vi "mqttTCPIPserver.vi"(0 "mqtt.lvclass":refnum<class "mqtt.lvclass">, 11 "error in (no error)":errorcluster) -> (4 "mqtt.lvclass 2":refnum<class "mqtt.lvclass">, 15 "error out":errorcluster)   [LabVIEW 2013, in "mqtt.lvclass"]
uses:
  mqtt.lvclass
  mqttTXqueue/mqttTXdataQueueFunction.ctl
  mqttTypedef/mqttQOSlevel.ctl
  mqttTypedef/mqttMessageType.ctl
  mqttTypedef/mqttFixedHeaderResponse.ctl
  mqttTypedef/mqttRXdataCluster.ctl
  mqttTXqueue/mqttRXsubscriptionEventFunction.ctl
  mqttTXqueue/mqttRXsubscriptionEventData.ctl
panel:
  out "rxCount":i32
  out "rxTelegram":u8[](array[numeric]) format="%02x"
  out "txError":errorcluster
  out "txTelegram":u8[](array[numeric]) format="%02x"
  out "payloadError":errorcluster
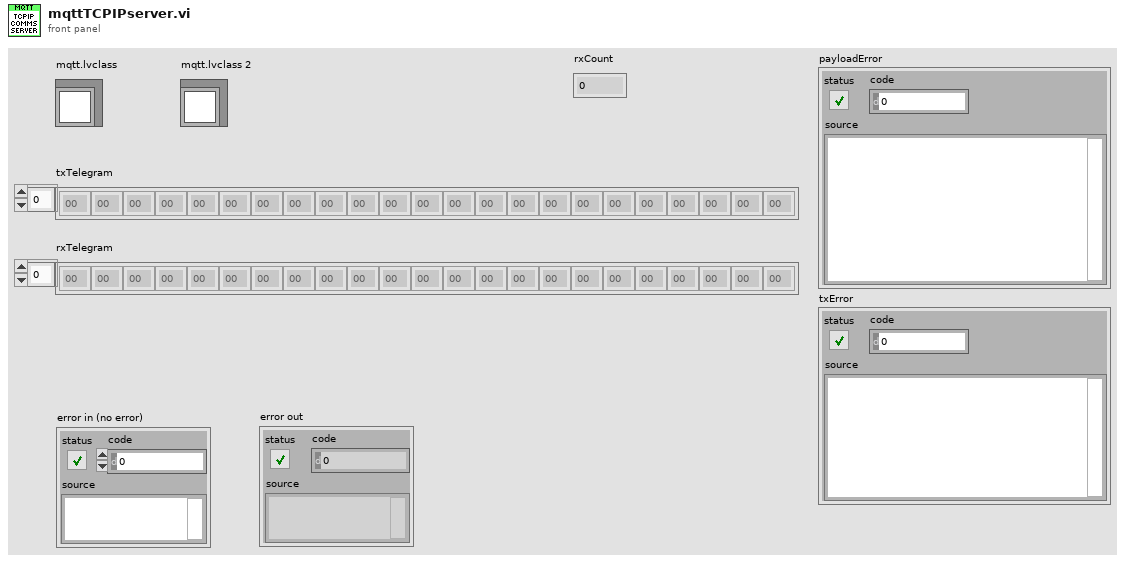
[diagram p1: front panel]
types:
  T1 = typedef "mqttTXdataQueueFunction.ctl" = enum16{"init", "deinit", "getQueue", "enqueue"}
  T2 = typedef "mqttRXdataCluster.ctl" = cluster{"fixedHdr":T3, "payload":u8[]}
  T3 = typedef "mqttFixedHeaderResponse.ctl" = cluster{"retain":bool, "qos":T4, "duplicate":bool, "response":T5}
  T4 = typedef "mqttQOSlevel.ctl" = enum8{"At most once", "At least once", "Exactly once", "Reserved"}
  T5 = typedef "mqttMessageType.ctl" = enum32{"Reserved", "CONNECT", "CONNACK", "PUBLISH", "PUBACK", "PUBREC", "PUBREL", "PUBCOMP", "SUBSCRIBE", "SUBACK", "UNSUBSCRIBE", "UNSUBACK", "PINGREQ", "PINGRESP", "DISCONNECT", "Reserved2"}
  T6 = typedef "mqttRXsubscriptionEventData.ctl" = cluster{"topic":string, "value":string, "messageID":u16}
  T7 = typedef "mqttRXsubscriptionEventFunction.ctl" = enum16{"init", "deinit", "getEventRef", "event"}
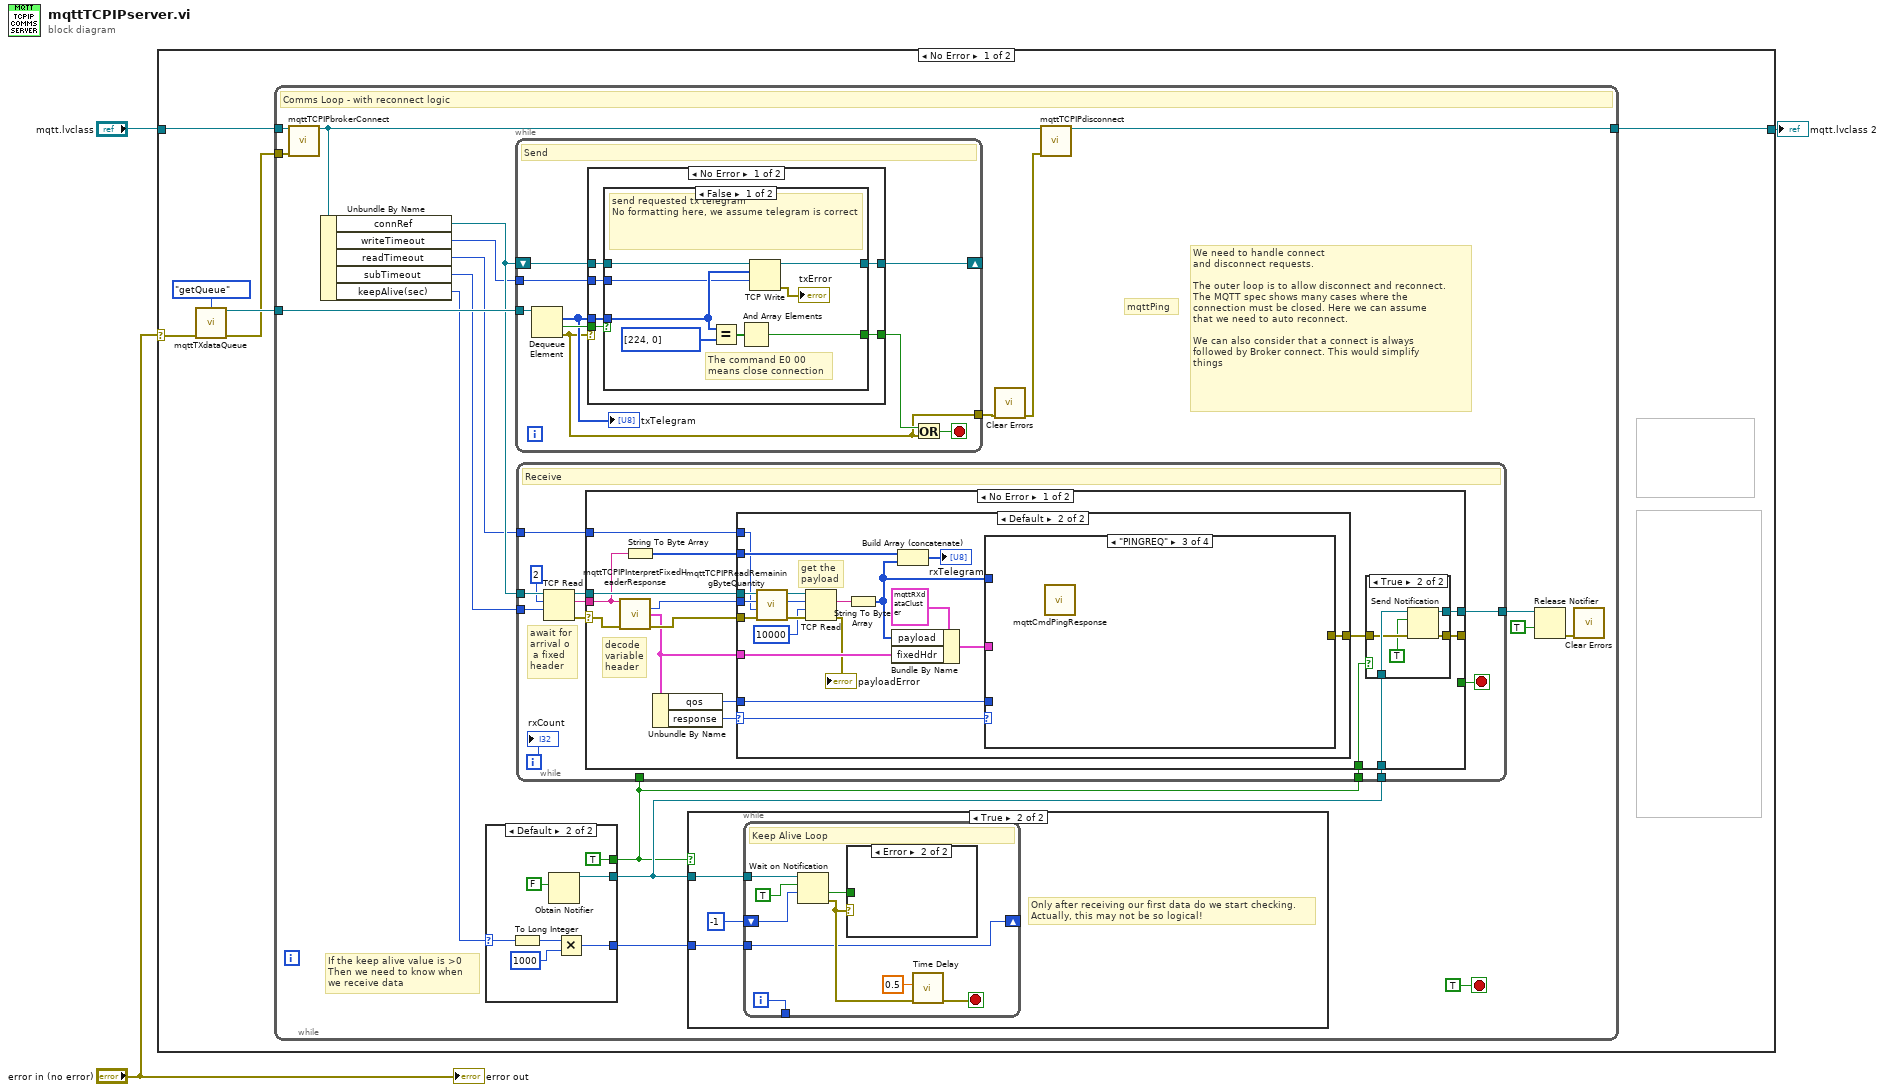
[diagram p0: block diagram]
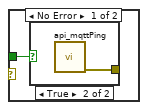
[diagram p3: hidden frame]
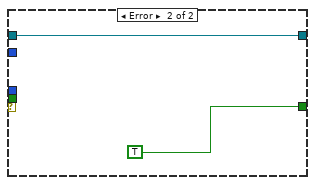
[diagram p7: hidden frame]
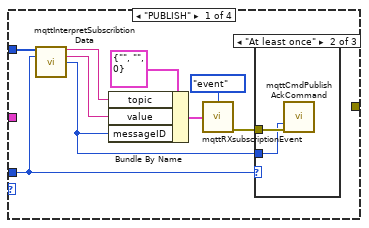
[diagram p10: hidden frame]
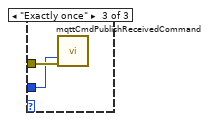
[diagram p12: hidden frame]
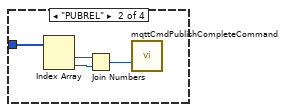
[diagram p13: hidden frame]
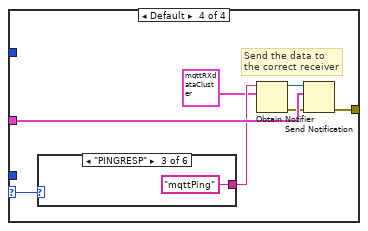
[diagram p14: hidden frame]
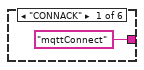
[diagram p15: hidden frame]
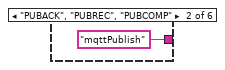
[diagram p16: hidden frame]
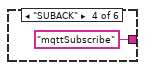
[diagram p17: hidden frame]
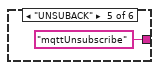
[diagram p18: hidden frame]
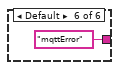
[diagram p19: hidden frame]
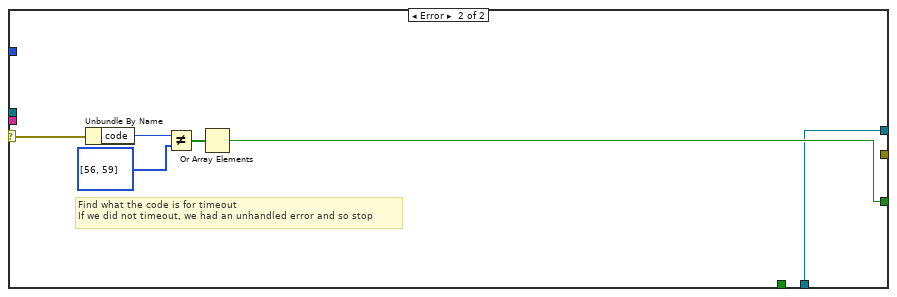
[diagram p20: hidden frame]
diagram:
  n1 = case shown="No Error" "error in (no error)" {
    selector: "error in (no error)" -> [w4 _]
    tunnel: "mqtt.lvclass" -> [w7 w163]
    tunnel: [w6 w163] -> w2
    frame No Error {
      n2 = call "mqttTXdataQueue.vi"("function"=mqttTXdataQueueFunction."getQueue", "error in (no error)"=w4) -> ("Queue out"=w9:refnum<queue>, "error out"=w5:errorcluster)  [unwired: 12 in]
      n3 = while {
        tunnel: w9 -> [w28]
        tunnel: w7 -> [w23]
        tunnel: [w21] -> w6
        tunnel: w5 -> [w22]
        stop <- TRUE stop-if-true
        # "If the keep alive value is >0\nThen we need to know when\nwe receive data"
        # "mqttPing"
        # "We need to handle connect\nand disconnect requests.\n\nThe outer loop is to allow disconnect and reconnect.\nThe MQTT spec shows many cases where the\nconnection must be closed. Here we can assume\nthat we need to auto reconnect.\n\nWe can also consider that a connect is always\nfollowed by Broker connect. This would simplify\nthings"
        # "Comms Loop - with reconnect logic"
        n4 = call "mqttTCPIPbrokerConnect.vi"("mqtt in"=w23, "error in (no error)"=w22) -> ("mqtt out"=w20:refnum<class "mqtt.lvclass">)  [unwired: 12 in, 1 out]
        n5 = Unbundle By Name(w20) -> ("connRef"=w26:refnum<k5>, "writeTimeout"=w19:i32, "readTimeout"=w18:i32, "subTimeout"=w17:i32, "keepAlive(sec)"=w11:u16)
        n6 = case shown="Default" w11 {
          selector: w11 -> [_ w44]
          tunnel: [_ w49] -> w16
          tunnel: [_ w45] -> w12
          tunnel: [_ TRUE] -> w10
          frame ..0 {
          }
          frame Default {
            n7 = To Long Integer(number=w44) -> (32bit integer=w47:i32)
            n8 = Obtain Notifier(notification data type=FALSE) -> (notifier out=w49:refnum<notifier>)  [unwired: 3 in, 2 out]
            n9 = Multiply(x=w47, y=1000) -> (x*y=w45:i32)
          }
        }
        n10 = while {
          tunnel: w28 -> [w58]
          shift-right: [w55] -> _
          shift-left: w26 -> [w56]
          tunnel: [w51] -> w25
          tunnel: w19 -> [w50]
          stop <- w54 stop-if-true
          # "Send"
          n11 = Dequeue Element(queue=w58) -> (element=w52:u8[], timed out?=w57:bool, error out=w51:errorcluster)  [unwired: 2 in, 1 out]
          "txTelegram" <- w52
          n12 = case shown="No Error" w51 {
            tunnel: w57 -> [w64 _]
            tunnel: w52 -> [w63 _]
            tunnel: w56 -> [w62 w75]
            tunnel: [w61 w75] -> w55
            tunnel: [w60 TRUE] -> w53
            tunnel: w50 -> [w59 _]
            frame No Error {
              n13 = case shown="False" w64 {
                tunnel: w63 -> [w70 _]
                tunnel: w62 -> [w72 w73]
                tunnel: [w71 w73] -> w61
                tunnel: [w67 _] -> w60
                tunnel: w59 -> [w65 _]
                frame False {
                  # "The command E0 00\nmeans close connection"
                  # "send requested tx telegram\nNo formatting here, we assume telegram is correct"
                  n14 = Equal?(x=w70, y=u8[] [224, 0] ("txTelegram 2")) -> (x = y?=w68:bool[])
                  n15 = And Array Elements(Boolean array=w68) -> (logical AND=w67:bool)
                  n16 = TCP Write(connection ID=w72, data in=w70, 9:w65) -> (connection ID out=w71:refnum<k5>, error out=→"txError":errorcluster)  [unwired: 1 in, 1 out]
                }
                frame True {
                  # "Queue Timed Out - do nothing.\nWe can later use this for the Keep Alive ping"
                }
              }
            }
            frame Error {
            }
          }
          n17 = Or(x=w53, y=w51) -> (x .or. y?=w54:bool)
        }
        n18 = while {
          tunnel: w26 -> [w87]
          tunnel: w18 -> [w80]
          tunnel: w17 -> [w79]
          tunnel: w16 -> [w78]
          tunnel: [w77] -> w15
          tunnel: w10 -> [w76]
          tunnel: w10 -> [_]
          i -> [w81]
          stop <- w82 stop-if-true
          # "await for\narrival o\n a fixed\nheader"
          # "Receive"
          n19 = TCP Read(connection ID=w87, bytes to read=2, 9:w79) -> (connection ID out=w86:refnum<k5>, data out=w83:string, error out=w85:errorcluster)  [unwired: 2 in]
          n20 = case shown="No Error" w85 {
            selector: w85 -> [w100 w162]
            tunnel: w86 -> [w101 _]
            tunnel: w83 -> [w96 _]
            tunnel: [_ w158] -> w82
            tunnel: w80 -> [w93 _]
            tunnel: w78 -> [w92 w157]
            tunnel: [w90 w157] -> w77
            tunnel: [w89 _] -> _
            tunnel: w76 -> [w88 _]
            frame No Error {
              # "decode\nvariable\nheader"
              n21 = call "mqttTCPIPInterpretFixedHeaderResponse.vi"("data in"=w96, "error in (no error)"=w100) -> ("remainingLengthByte1"=w102:u8, "output cluster"=w98:T3, "error out"=w99:errorcluster)  [unwired: 11 in]
              n22 = String To Byte Array(string=w96) -> (unsigned byte array=w95:u8[])
              n23 = Unbundle By Name(w98) -> ("qos"=w94:T4, "response"=w97:T5)
              n24 = case shown="Default" w97 {
                selector: w97 -> [_ w116]
                tunnel: w102 -> [_ w126]
                tunnel: w101 -> [_ w125]
                tunnel: w99 -> [_ w118]
                tunnel: w98 -> [_ w117]
                tunnel: w95 -> [_ w113]
                tunnel: w94 -> [_ w112]
                tunnel: w93 -> [_ w109]
                tunnel: [_ w108] -> w91
                frame "CONNECT", "SUBSCRIBE" {
                  # "The client should not receive these commands.\nI had some problems with these commands being received\nand it appears this was a broker issue. However, to ignore\nmessages that we should not receive is no bad thing."
                }
                frame Default {
                  # "get the\npayload"
                  n25 = call "mqttTCPIPReadRemainingByteQuantity.vi"("error in (no error)"=w118, "readTimeout ms (2000)"=w109, "remainingLengthByte1"=w126, "connRef in"=w125) -> ("error out"=w123:errorcluster, "remainingLength"=w122:i32, "connRef out"=w124:refnum<k5>)  [unwired: 5 in]
                  n26 = TCP Read(connection ID=w124, bytes to read=w122, error in (no error)=w123, 9:10000 ("timeout ms (25000)")) -> (data out=w120:string, error out=→"payloadError":errorcluster)  [unwired: 1 in, 1 out]
                  n27 = String To Byte Array(string=w120) -> (unsigned byte array=w110:u8[])
                  n28 = Bundle By Name(cluster=T2 {"fixedHdr"={"retain"=FALSE, "qos"=enum."At most once", "duplicate"=FALSE, "response"=enum."Reserved"}, "payload"=[]} ("output cluster"), "payload"=w110, "fixedHdr"=w117) -> (w114:T2)
                  n29 = Build Array (concatenate)(w113, w110) -> (→"rxTelegram":u8[])
                  n30 = case shown="\"PINGREQ\"" w116 {
                    selector: w116 -> [_ _ _ w150]
                    tunnel: w114 -> [_ _ _ w149]
                    tunnel: w112 -> [w128 _ _ _]
                    tunnel: w110 -> [w132 w143 _ _]
                    tunnel: [_ _ _ w144] -> w108
                    frame "PUBLISH" {
                      n31 = call "mqttInterpretSubscribtionData.vi"("rxTelegram in"=w132, "qos"=w128) -> ("topic"=w131:string, "value"=w130:string, "messageID"=w127:u16)  [unwired: 10 in, 1 out]
                      n32 = Bundle By Name(cluster=T6 {"topic"="", "value"="", "messageID"=0} ("data"), "topic"=w131, "value"=w130, "messageID"=w127) -> (w133:T6)
                      n33 = call "mqttRXsubscriptionEvent.vi"("function"=mqttRXsubscriptionEventFunction."event", "data"=w133) -> ("error out"=w129:errorcluster)  [unwired: 12 in, 1 out]
                      n34 = case shown="\"At least once\"" w128 {
                        tunnel: w129 -> [_ w137 w139]
                        tunnel: w127 -> [_ w136 w138]
                        frame Default {
                        }
                        frame "At least once" {
                          n35 = call "mqttCmdPublishAckCommand.vi"("messageID"=w136, "error in (no error)"=w137) -> ()  [unwired: 13 in, 1 out]
                        }
                        frame "Exactly once" {
                          n36 = call "mqttCmdPublishReceivedCommand.vi"("messageID"=w138, "error in (no error)"=w139) -> ()  [unwired: 13 in, 1 out]
                        }
                      }
                    }
                    frame "PUBREL" {
                      n37 = Index Array(array=w143) -> (element #1=w142:u8, element #2=w141:u8)  [unwired: 2 in]
                      n38 = Join Numbers(hi=w142, lo=w141) -> ((hi.lo)=w140:u16)
                      n39 = call "mqttCmdPublishCompleteCommand.vi"("messageID"=w140) -> ()  [unwired: 14 in, 1 out]
                    }
                    frame "PINGREQ" {
                      n40 = call "mqttCmdPingResponse.vi"() -> ()  [unwired: 15 in, 1 out]
                    }
                    frame Default {
                      # "Send the data to\nthe correct receiver"
                      n41 = case shown="\"PINGRESP\"" w150 {
                        tunnel: ["mqttConnect" ("name (unnamed)") "mqttPublish" ("name (unnamed)") "mqttPing" ("name (unnamed)") "mqttSubscribe" ("name (unnamed)") "mqttUnsubscribe" ("name (unnamed)") "mqttError" ("name (unnamed)")] -> w148
                        frame "CONNACK" {
                        }
                        frame "PUBACK", "PUBREC", "PUBCOMP" {
                        }
                        frame "PINGRESP" {
                        }
                        frame "SUBACK" {
                        }
                        frame "UNSUBACK" {
                        }
                        frame Default {
                        }
                      }
                      n42 = Obtain Notifier(name (unnamed)=w148, notification data type=T2 {"fixedHdr"={"retain"=FALSE, "qos"=enum."At most once", "duplicate"=FALSE, "response"=enum."Reserved"}, "payload"=[]} ("output cluster")) -> (notifier out=w147:refnum<notifier>, error out=w145:errorcluster)  [unwired: 2 in, 1 out]
                      n43 = Send Notification(notification=w149, notifier=w147, error in (no error)=w145) -> (error out=w144:errorcluster)  [unwired: 1 out]
                    }
                  }
                }
              }
              n44 = case shown="True" w88 {
                tunnel: w92 -> [_ w107]
                tunnel: w91 -> [_ w106]
                tunnel: [_ w104] -> w90
                tunnel: [_ w103] -> w89
                frame False {
                }
                frame True {
                  n45 = Send Notification(notification=TRUE, notifier=w107, error in (no error)=w106) -> (notifier out=w104:refnum<notifier>, error out=w103:errorcluster)
                }
              }
            }
            frame Error {
              # "Find what the code is for timeout\nIf we did not timeout, we had an unhandled error and so stop"
              n46 = Unbundle By Name(w162) -> ("code"=w161:i32)
              n47 = Not Equal?(x=w161, y=i32[] [56, 59]) -> (x != y?=w159:bool[])
              n48 = Or Array Elements(Boolean array=w159) -> (logical OR=w158:bool)
            }
          }
          "rxCount" <- w81
        }
        n49 = case shown="True" w10 {
          tunnel: w16 -> [_ w31]
          tunnel: w12 -> [_ w30]
          frame False {
          }
          frame True {
            # "Only after receiving our first data do we start checking.\nActually, this may not be so logical!"
            n50 = while {
              tunnel: w31 -> [w40]
              tunnel: [w35] -> _
              shift-right: [w32] -> _
              shift-left: -1 -> [w39]
              tunnel: w30 -> [w32]
              i -> [w35]
              stop <- w36 stop-if-true
              # "Keep Alive Loop"
              n51 = Wait on Notification(notifier=w40, ignore previous (F)=TRUE, timeout in ms (-1)=w39) -> (timed out?=w38:bool, error out=w33:errorcluster)  [unwired: 1 in, 2 out]
              n52 = case shown="Error" w33 {
                tunnel: w38 -> [w41 _]
                frame No Error {
                  n53 = case shown="True" w41 {
                    tunnel: [_ w42] -> _
                    frame False {
                    }
                    frame True {
                      n54 = call "api_mqttPing.vi"() -> ("error out"=w42:errorcluster)  [unwired: 14 in, 1 out]
                    }
                  }
                }
                frame Error {
                }
              }
              n55 = call "Time Delay"("error in (no error)"=w33, "Delay Time (s)"=0.5) -> ("error out"=w36:errorcluster)  [unwired: 9 in]
            }
          }
        }
        n56 = call <vilib>:"Clear Errors.vi"("error in (no error)"=w25) -> ("error out"=w24:errorcluster)  [unwired: 5 in, 1 out]
        n57 = call "mqttTCPIPdisconnect.vi"("mqtt in"=w20, "error in (no error)"=w24) -> ("mqtt out"=w21:refnum<class "mqtt.lvclass">)  [unwired: 12 in, 1 out]
        n58 = Release Notifier(notifier=w15, force destroy? (F)=TRUE) -> (error out=w13:errorcluster)  [unwired: 1 in, 2 out]
        n59 = call <vilib>:"Clear Errors.vi"("error in (no error)"=w13) -> ()  [unwired: 5 in, 2 out]
      }
    }
    frame Error {
    }
  }
  "mqtt.lvclass 2" <- w2
  "error out" <- "error in (no error)"
